vi "AssignToConnPane.vi"(6 "recommended":bool, 8 "error in (no error)":errorcluster, 9 "term index":u32, 10 "Control":refnum<vi>, 11 "vi reference":refnum<vi>) -> (0 "error out":errorcluster)   [LabVIEW 2017, in "MessageGen.lvlib"]
uses:
  <vilib>/addons/InsightCM/MessageBus/CodeGen/MessageGen.lvlib
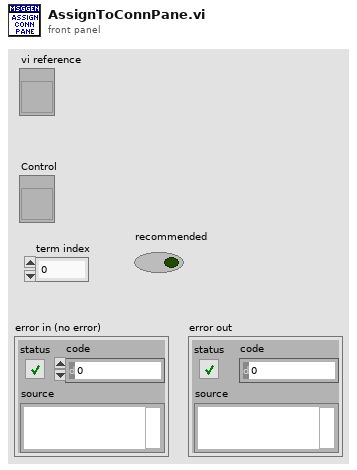
[diagram p1: front panel]
types:
  T1 = enum16{"Invalid Wire Rule", "Required", "Recommended", "Optional", "Dynamic Dispatch"}
  T2 = enum16{"Invalid Wire Rule", "Required", "Recommended", "Optional", "Dynamic Dispatch"}[]
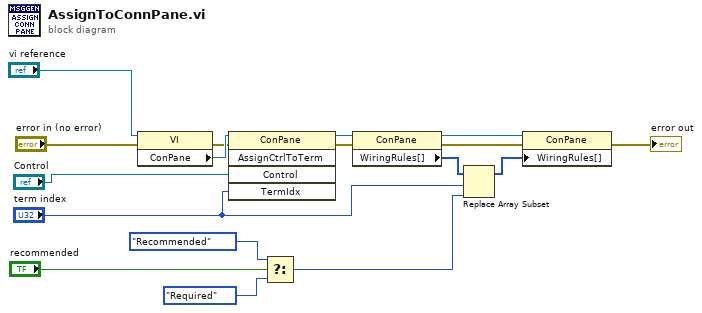
[diagram p0: block diagram]
diagram:
  n1 = property class="VI"(reference="vi reference", error in="error in (no error)") -> (error out=w16:errorcluster, "ConPane"=w17:refnum<vi>)  [unwired: 1 out]
  n2 = invoke class="ConPane" method="AssignCtrlToTerm"(reference=w17, error in=w16, "Control"="Control", "TermIdx"="term index") -> (reference out=w15:refnum<vi>, error out=w14:errorcluster)  [unwired: 1 in, 3 out]
  n3 = Select(t=T1."Recommended" ("new element/subarray"), s="recommended", f=T1."Required" ("new element/subarray")) -> (s? t:f=w2:T1)
  n4 = property class="ConPane"(reference=w15, error in=w14) -> (reference out=w13:refnum<vi>, error out=w12:errorcluster, "WiringRules[]"=w11:T2)
  n5 = Replace Array Subset(array=w11, new element=w2, index="term index") -> (w10:T2)
  n6 = property class="ConPane"(reference=w13, error in=w12, "WiringRules[]"=w10) -> (error out=→"error out":errorcluster)  [unwired: 1 out]
